vi "Teleop.vi"(10 "Match Info":T1={"Autonomous Elapsed Seconds"=0.0, "TeleOp Elapsed Seconds"=0.0, "Disabled Elapsed Seconds"=0.0, "Visited Autonomous"=FALSE, "Visited TeleOp"=FALSE, "Visited Disabled"=FALSE, "Autonomous Settings"={"Autonomous Style"=enum."Independent", "VI Refnum"=refnum}}, 11 "Call Context":T2) -> ()   [LabVIEW 2019]
doc: "This VI is called for each TeleOp packet received from the DS where the robot is not disabled. It is often used to read from the joysticks and update I/O or to update setpoints for timed control loops. It should complete and return within 20 milliseconds or it may miss DS packets."
uses:
  <vilib>/Rock Robotics/WPI/DriverStation/WPI_DriverStationDerivedRobotMode.ctl
  <vilib>/Rock Robotics/WPI/DriverStation/WPI_DriverStationMatch Info.ctl
  <vilib>/Rock Robotics/WPI/Utilities/WPI_GetSetVariantRefNum.vi
  Axes_n_Buttons_Global.vi
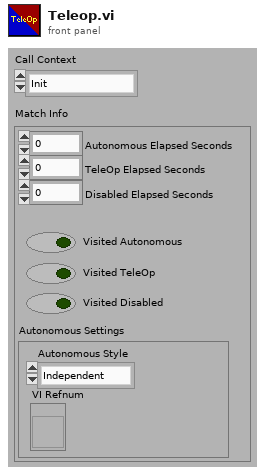
[diagram p1: front panel]
types:
  T1 = typedef "WPI_DriverStationMatch Info.ctl" = cluster{"Autonomous Elapsed Seconds":dbl, "TeleOp Elapsed Seconds":dbl, "Disabled Elapsed Seconds":dbl, "Visited Autonomous":bool, "Visited TeleOp":bool, "Visited Disabled":bool, "Autonomous Settings":cluster{"Autonomous Style":enum16{"Iterative", "Independent"}, "VI Refnum":refnum<vi>}}
  T2 = typedef "WPI_DriverStationDerivedRobotMode.ctl" = enum16{"Init", "Execute", "Stop"}
  T3 = typedef "WPI_JoystickDevRef.ctl" = cluster{"Device":T4}
  T4 = typedef "WPI_JoystickDeviceEnum.ctl" = enum16{"USB 0", "USB 1", "USB 2", "USB 3", "USB 4", "USB 5"}
  T5 = typedef "D-Pad.ctl" = cluster{"Top":bool, "Bottom":bool, "None":bool, "Right":bool, "Left":bool}
  T6 = typedef "Axes Cluster.ctl" = cluster{"Axes[0]":dbl, "Axes[1]":dbl, "Axes[2]":dbl, "Axes[3]":dbl, "Axes[4]":dbl, "Axes[5]":dbl, "Axes[6]":dbl, "Axes[7]":dbl, "Axes[8]":dbl}
  T7 = typedef "Button Cluster.ctl" = cluster{"Buttons[0]":bool, "Buttons[1]":bool, "Buttons[2]":bool, "Buttons[3]":bool, "Buttons[4]":bool, "Buttons[5]":bool, "Buttons[6]":bool, "Buttons[7]":bool, "Buttons[8]":bool, "Buttons[9]":bool}
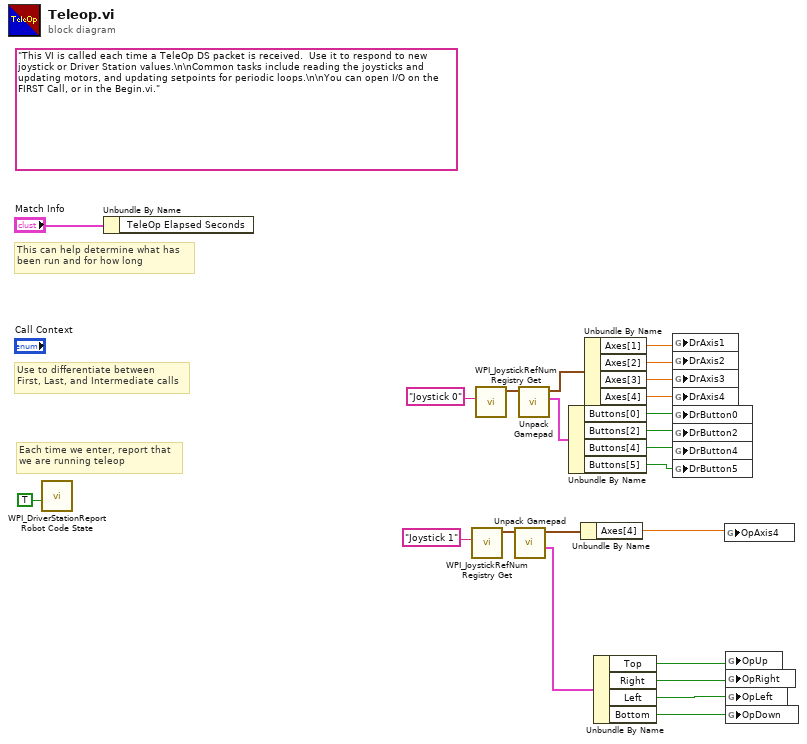
[diagram p0: block diagram]
diagram:
  (unwired) "This VI is called each time a TeleOp DS packet is received.  Use it to respond to new joystick or Driver Station values.\n\nCommon tasks include reading the joysticks and updating motors, and updating setpoints for periodic loops.\n\nYou can open I/O on the FIRST Call, or in the Begin.vi."
  # "Each time we enter, report that\nwe are running teleop"
  # "Use to differentiate between\nFirst, Last, and Intermediate calls"
  # "This can help determine what has\nbeen run and for how long"
  n1 = call <vilib>:"WPI_DriverStationReport Robot Code State.vi"("TeleOp"=TRUE ("Autonomous")) -> ()  [unwired: 10 in, 1 out]
  n2 = Unbundle By Name("Match Info") -> ()  [unwired: 1 out]
  n3 = call <vilib>:"WPI_JoystickRefNum Registry Get.vi"("refnum name"="Joystick 1") -> ("JoystickDevRef"=w9:T3)  [unwired: 1 in, 9 out]
  n4 = call <vilib>:"WPI_JoystickRefNum Registry Get.vi"("refnum name"="Joystick 0") -> ("JoystickDevRef"=w20:T3)  [unwired: 1 in, 9 out]
  n5 = call "Unpack Gamepad.vi"("JoystickDevRef"=w9) -> ("D-Pad"=w7:T5, "Axes"=w2:T6)  [unwired: 8 in, 1 out]
  n6 = call "Unpack Gamepad.vi"("JoystickDevRef"=w20) -> ("Button Cluster"=w18:T7, "Axes"=w19:T6)  [unwired: 8 in, 1 out]
  n7 = Unbundle By Name(w18) -> ("Buttons[0]"=w13:bool, "Buttons[2]"=w12:bool, "Buttons[4]"=w11:bool, "Buttons[5]"=w10:bool)
  n8 = Unbundle By Name(w2) -> ("Axes[4]"=w1:dbl)
  n9 = Unbundle By Name(w19) -> ("Axes[1]"=w17:dbl, "Axes[2]"=w16:dbl, "Axes[3]"=w15:dbl, "Axes[4]"=w14:dbl)
  n10 = Unbundle By Name(w7) -> ("Top"=w6:bool, "Right"=w5:bool, "Left"=w4:bool, "Bottom"=w3:bool)
  n11 = global write "Axes_n_Buttons_Global.vi" "DrAxis1"(w17) -> ()
  n12 = global write "Axes_n_Buttons_Global.vi" "DrAxis2"(w16) -> ()
  n13 = global write "Axes_n_Buttons_Global.vi" "DrAxis3"(w15) -> ()
  n14 = global write "Axes_n_Buttons_Global.vi" "DrAxis4"(w14) -> ()
  n15 = global write "Axes_n_Buttons_Global.vi" "DrButton0"(w13) -> ()
  n16 = global write "Axes_n_Buttons_Global.vi" "DrButton2"(w12) -> ()
  n17 = global write "Axes_n_Buttons_Global.vi" "DrButton4"(w11) -> ()
  n18 = global write "Axes_n_Buttons_Global.vi" "DrButton5"(w10) -> ()
  n19 = global write "Axes_n_Buttons_Global.vi" "OpAxis4"(w1) -> ()
  n20 = global write "Axes_n_Buttons_Global.vi" "OpUp"(w6) -> ()
  n21 = global write "Axes_n_Buttons_Global.vi" "OpRight"(w5) -> ()
  n22 = global write "Axes_n_Buttons_Global.vi" "OpLeft"(w4) -> ()
  n23 = global write "Axes_n_Buttons_Global.vi" "OpDown"(w3) -> ()
